vi "CloseFile.vi"(8 "error in (no error)":errorcluster, 11 "ReadWrite in":refnum<class "ReadWrite.lvclass">) -> (0 "error out":errorcluster)   [LabVIEW 2021, in "ReadWrite.lvclass"]
uses:
  ReadWrite.lvclass
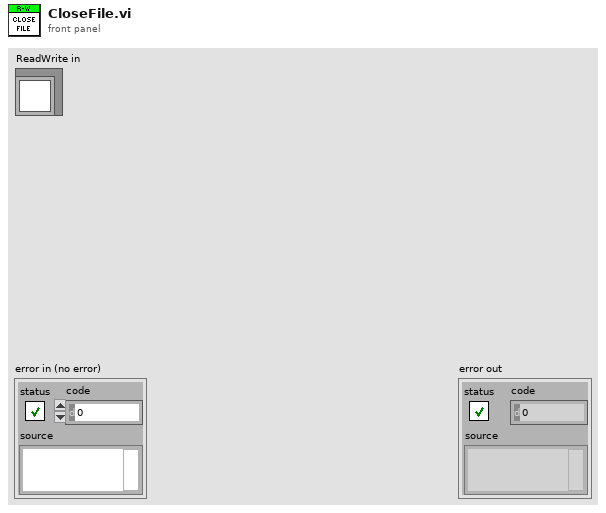
[diagram p1: front panel]
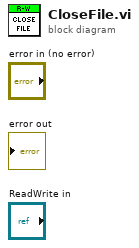
[diagram p0: block diagram]
diagram:
